vi "Server Routing Loop.vi"(8 "error in (no error)":errorcluster, 11 "TCPMessaging in":refnum<class "TCPMessaging.lvclass">) -> (0 "error out":errorcluster)   [LabVIEW 2020, in "Vecto.lvlib" / "TCPMessaging.lvclass"]
doc: "Routes outgoing payloads to the correct client."
uses:
  TCPMessaging.lvclass
  Target Group Maps.ctl
  TCPMessaging.lvclass/TCPMessaging.ctl
  SequenceCountService/SequenceCountService.lvclass/SequenceCountService.ctl
  lv-promises/Promises/Promise/Promise.lvclass
  SequenceCountService/SequenceCountService.lvclass
  proto/TcpPayload/TcpPayload.lvlib
  Vecto.lvlib
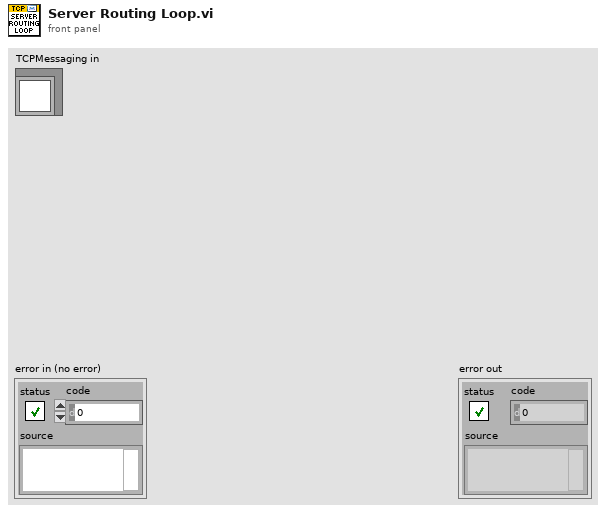
[diagram p1: front panel]
types:
  T1 = typedef "Vecto.lvlib/TCPMessaging.lvclass/Target Group Maps.ctl" = cluster{"Target":map{u32, u32[]}, "Node":map{u32, u32[]}}
  T2 = typedef "Vecto.lvlib/TX Payload.ctl" = cluster{"Target ID":u32, "Payload":string}
  T3 = typedef "Vecto.lvlib/Send Message Data.ctl" = cluster{"TcpPayload":T4, "Register Reply":bool, "Reply Promise":refnum<class "Promise.lvclass">, "Reply Deadline":dbl}
  T4 = typedef "TcpPayload.lvlib/Data.ctl" = cluster{"target_node":u32, "source_id":u32, "sequence":u32, "timestamp":i64, "type":string, "task_id":string, "payload":u8[]}
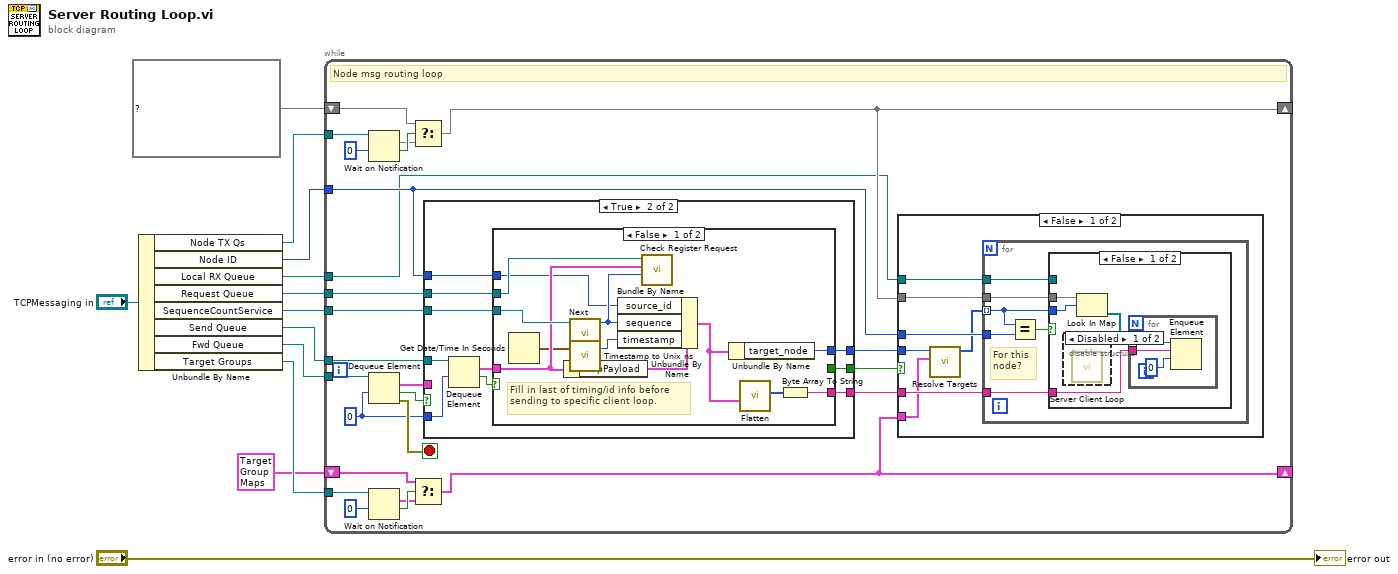
[diagram p0: block diagram]
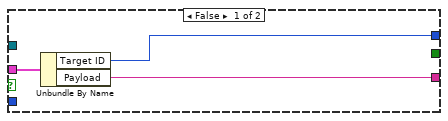
[diagram p2: hidden frame]
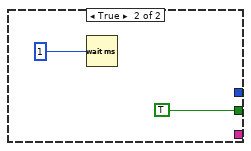
[diagram p3: hidden frame]
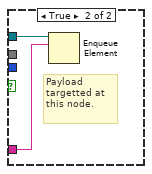
[diagram p5: hidden frame]
diagram:
  n1 = Unbundle By Name("TCPMessaging in") -> ("Node TX Qs"=w3:refnum<notifier>, "Node ID"=w4:u32, "Local RX Queue"=w2:refnum<queue>, "Request Queue"=w7:refnum<queue>, "SequenceCountService"=w8:refnum<class "SequenceCountService.lvclass">, "Send Queue"=w11:refnum<queue>, "Fwd Queue"=w9:refnum<queue>, "Target Groups"=w6:refnum<notifier>)
  n2 = while {
    tunnel: w11 -> [w36]
    tunnel: w3 -> [w35]
    shift-right: [w24] -> _
    shift-left: map{u32, refnum<queue>[]} {} ("notification") -> [w32]
    tunnel: w9 -> [w31]
    tunnel: w8 -> [w26]
    tunnel: w2 -> [w14]
    tunnel: w7 -> [w22]
    tunnel: w6 -> [w21]
    shift-right: [w16] -> _
    shift-left: T1 {"Target"={}, "Node"={}} ("Target Group Maps") -> [w17]
    tunnel: w4 -> [w15]
    stop <- w37 stop-if-true
    w30 = 0 ("timeout in ms (-1)")
    # "Node msg routing loop"
    n3 = Wait on Notification(notifier=w35, timeout in ms (-1)=0) -> (notification=w13:map{u32, refnum<queue>[]}, timed out?=w33:bool)  [unwired: 2 in, 2 out]
    n4 = Dequeue Element(queue=w31, timeout in ms (-1)=w30) -> (element=w28:T2, timed out?=w29:bool, error out=w37:errorcluster)  [unwired: 1 in, 1 out]
    n5 = Wait on Notification(notifier=w21, timeout in ms (-1)=0) -> (notification=w18:T1, timed out?=w19:bool)  [unwired: 2 in, 2 out]
    n6 = Select(t=w32, s=w33, f=w13) -> (s? t:f=w24:map{u32, refnum<queue>[]})
    n7 = Select(t=w17, s=w19, f=w18) -> (s? t:f=w16:T1)
    n8 = case shown="True" w29 {
      tunnel: w36 -> [_ w50]
      tunnel: w30 -> [_ w48]
      tunnel: w28 -> [w40 _]
      tunnel: [w39 w43] -> w27
      tunnel: w15 -> [_ w46]
      tunnel: w26 -> [_ w45]
      tunnel: [w38 w44] -> w25
      tunnel: [_ w42] -> w23
      tunnel: w22 -> [_ w41]
      frame False {
        n9 = Unbundle By Name(w40) -> ("Target ID"=w39:u32, "Payload"=w38:string)
      }
      frame True {
        n10 = Dequeue Element(queue=w50, timeout in ms (-1)=w48) -> (element=w49:T3, timed out?=w47:bool)  [unwired: 1 in, 2 out]
        n11 = case shown="False" w47 {
          tunnel: w49 -> [w54 _]
          tunnel: w46 -> [w52 _]
          tunnel: w45 -> [w62 _]
          tunnel: [w60 _] -> w44
          tunnel: [w57 _] -> w43
          tunnel: [_ TRUE] -> w42
          tunnel: w41 -> [w53 _]
          frame False {
            # "Fill in last of timing/id info before sending to specific client loop."
            n12 = Get Date/Time In Seconds() -> (seconds since 1Jan1904=w51:timestamp)
            n13 = Unbundle By Name(w54) -> ("TcpPayload"=w56:T4)
            n14 = call "Next.vi"("SequenceCountService in"=w62) -> ("Sequence"=w55:u32)  [unwired: 9 in, 1 out]
            n15 = call "Timestamp to Unix ns.vi"("Time Stamp"=w51) -> ("unix ns"=w61:i64)  [unwired: 2 in]
            n16 = Bundle By Name(cluster=w56, "source_id"=w52, "sequence"=w55, "timestamp"=w61) -> (w58:T4)
            n17 = call "Check Register Request.vi"("Sequence"=w55, "Send Message Data"=w54, "Request Queue"=w53) -> ()  [unwired: 8 in, 1 out]
            n18 = Unbundle By Name(w58) -> ("target_node"=w57:u32)
            n19 = call "Flatten.vi"("Data"=w58) -> ("Buffer"=w59:u8[])  [unwired: 9 in, 1 out]
            n20 = Byte Array To String(unsigned byte array=w59) -> (string=w60:string)
          }
          frame True {
            n21 = Wait (ms)(milliseconds to wait=u32 1) -> ()  [unwired: 1 out]
          }
        }
      }
    }
    n22 = case shown="False" w23 {
      tunnel: w27 -> [w66 _]
      tunnel: w25 -> [w71 _]
      tunnel: w24 -> [w70 _]
      tunnel: w16 -> [w67 _]
      tunnel: w15 -> [w69 _]
      tunnel: w14 -> [w68 _]
      frame False {
        n23 = call "Resolve Targets.vi"("Target Group Maps"=w67, "Target ID"=w66) -> ("Targets"=w65:u32[])  [unwired: 9 in]
        n24 = for {
          tunnel: w65 -> [w74] mode=indexing
          tunnel: w71 -> [w76]
          tunnel: w70 -> [w77]
          tunnel: w69 -> [w75]
          tunnel: w68 -> [w72]
          # "For this node?"
          n25 = Equal?(x=w74, y=w75) -> (x = y?=w73:bool)
          n26 = case shown="False" w73 {
            tunnel: w77 -> [w80 _]
            tunnel: w76 -> [w81 w85]
            tunnel: w74 -> [w79 _]
            tunnel: w72 -> [_ w86]
            frame False {
              n27 = disable-structure shown="Disabled" {
                frame Disabled {
                  n28 = call "Server Client Loop.vi"() -> ()  [unwired: 12 in]
                }
                frame Enabled {
                }
              }
              n29 = Look In Map(map=w80, key=w79) -> (value=w78:refnum<queue>[])  [unwired: 1 in, 1 out]
              n30 = for {
                tunnel: w81 -> [w84]
                tunnel: w78 -> [w82] mode=indexing
                n31 = Enqueue Element(queue=w82, element=w84, timeout in ms (-1)=0) -> ()  [unwired: 1 in, 3 out]
              }
            }
            frame True {
              # "Payload targetted at this node."
              n32 = Enqueue Element(queue=w86, element=w85) -> ()  [unwired: 2 in, 3 out]
            }
          }
        }
      }
      frame True {
        # "Sending message is skipped"
      }
    }
  }
  "error out" <- "error in (no error)"
